vi "Simulation Lab signal B220061.vi"() -> ()   [LabVIEW 2020]
panel:
  out "Waveform Graph 2":dynamicdata(graph)
  out "Waveform Graph":dynamicdata(graph)
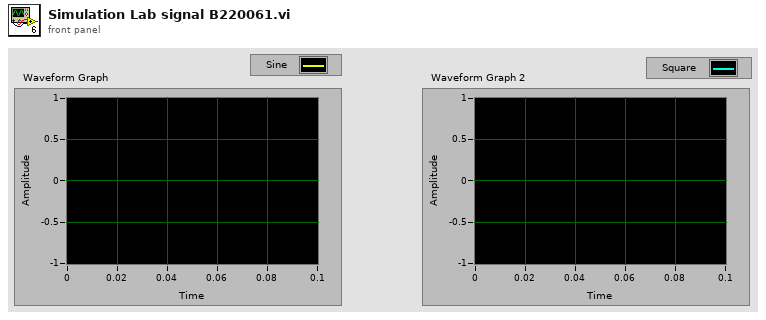
[diagram p1: front panel]
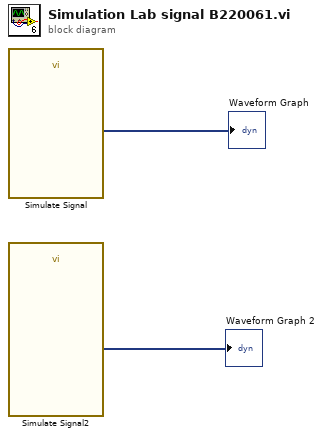
[diagram p0: block diagram]
diagram:
  n1 = call "Simulate Signal"() -> ("Sine"=→"Waveform Graph":dynamicdata)  [unwired: 14 in, 1 out]
  n2 = call "Simulate Signal2"() -> ("Square"=→"Waveform Graph 2":dynamicdata)  [unwired: 14 in, 1 out]
